vi "Three Pins Logic Gate Demo.vi"(1 "Pin2":bool, 2 "Pin1":bool, 3 "Pin0":bool) -> (0 "Output":bool)   [LabVIEW 2012]
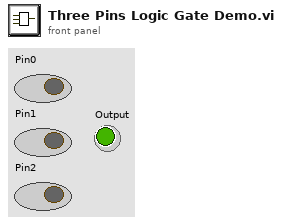
[diagram p1: front panel]
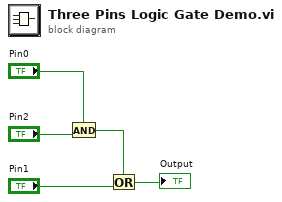
[diagram p0: block diagram]
diagram:
  n1 = And(x="Pin0", y="Pin2") -> (x .and. y?=w3:bool)
  n2 = Or(x=w3, y="Pin1") -> (x .or. y?=→"Output":bool)
